vi "_PC_RTLoop_ReadLaserStatus.vi"(8 "error in (no error)":errorcluster, 9 "LaserStatus_string_reference in":refnum<vi>, 10 "Laser Status byte":refnum<vi>, 11 "stopRefnum":refnum<vi>) -> (0 "error out":errorcluster)   [LabVIEW 2018]
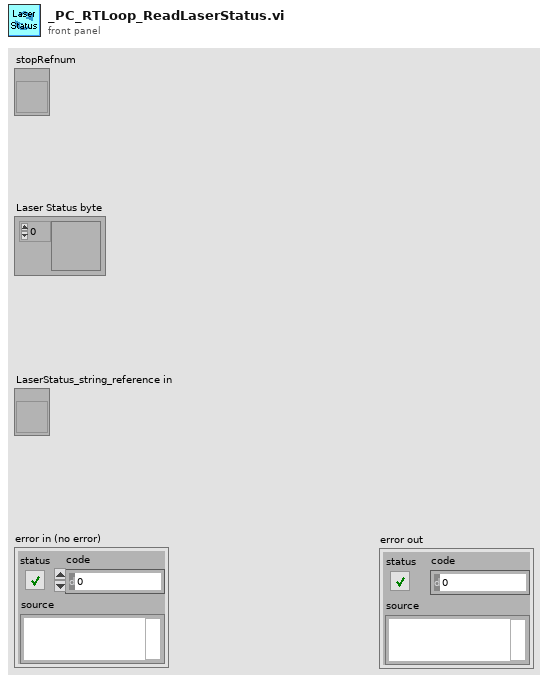
[diagram p1: front panel]
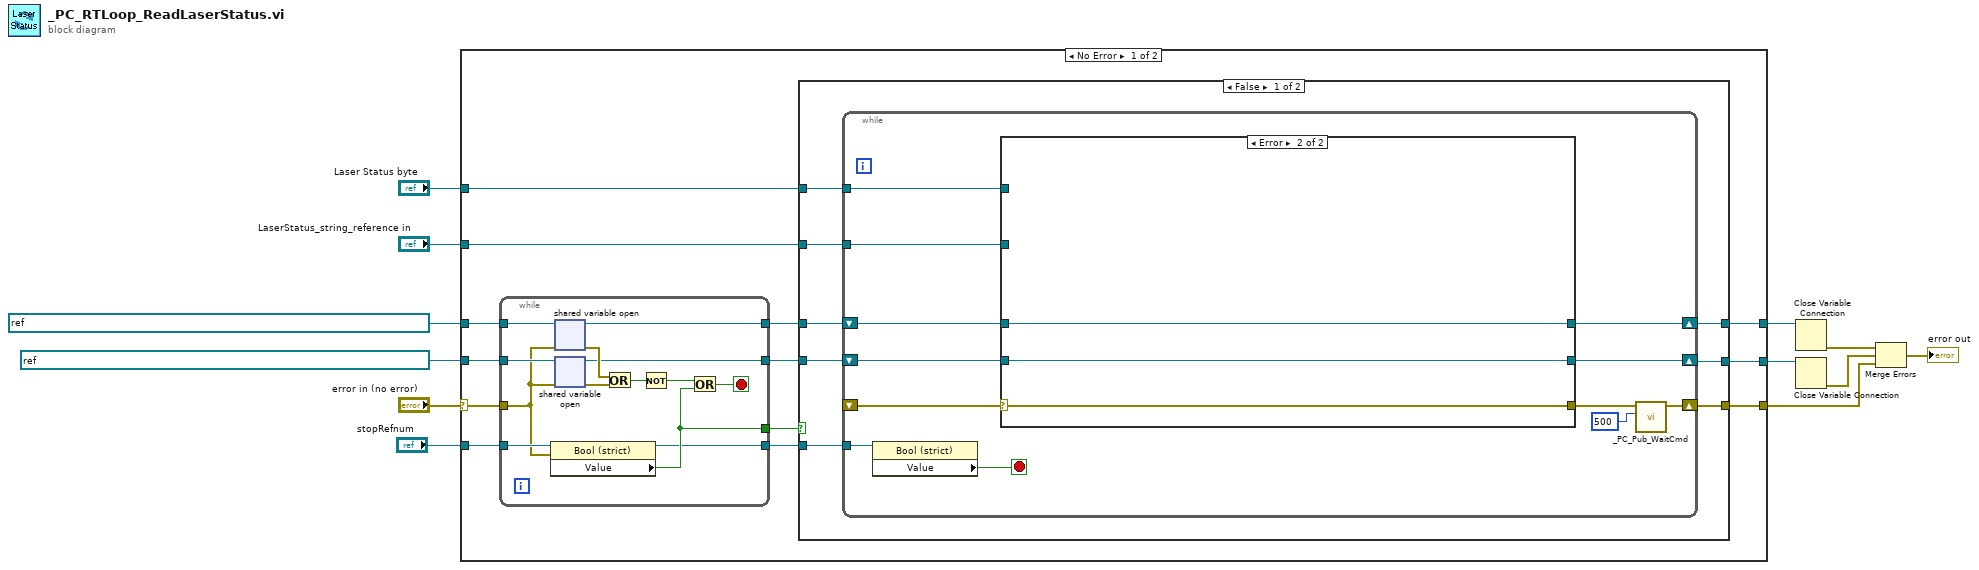
[diagram p0: block diagram]
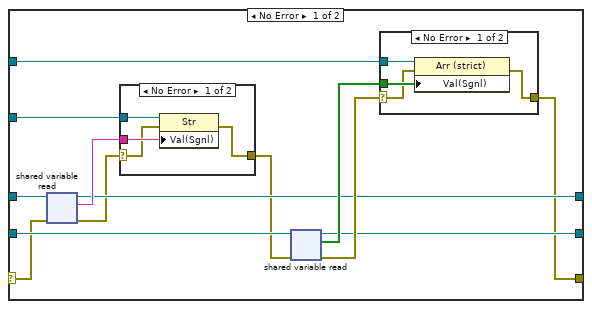
[diagram p2: hidden frame]
diagram:
  n1 = case shown="No Error" "error in (no error)" {
    selector: "error in (no error)" -> [w23 w87]
    tunnel: refnum<k21> "ni.var.psp://NI-sbRIO/_RT_CtrlLoop_Laser_Variables/LaserStatus_string" ("shared variable refnum in") -> [w25 w89]
    tunnel: refnum<k21> "ni.var.psp://NI-sbRIO/_RT_CtrlLoop_Laser_Variables/LaserStatusByte" ("shared variable refnum in") -> [w24 w88]
    tunnel: "LaserStatus_string_reference in" -> [w20 _]
    tunnel: "Laser Status byte" -> [w19 _]
    tunnel: [w18 w89] -> w7
    tunnel: [w17 w88] -> w6
    tunnel: "stopRefnum" -> [w16 _]
    tunnel: [w13 w87] -> w2
    frame No Error {
      n2 = while {
        tunnel: w25 -> [w86]
        tunnel: w24 -> [w85]
        tunnel: w23 -> [w74]
        tunnel: [w81] -> w21
        tunnel: [w80] -> w22
        tunnel: w16 -> [w77]
        tunnel: [w76] -> w14
        tunnel: [w75] -> w15
        stop <- w78 stop-if-true
        n3 = property class="Bool (strict)"(reference=w77, error in=w74) -> (reference out=w75:refnum<vi>, "Value"=w76:bool)  [unwired: 1 out]
        n4 = shared-variable-open(w86, w74) -> (w80:refnum<k21>, w84:errorcluster)
        n5 = shared-variable-open(w85, w74) -> (w81:refnum<k21>, w83:errorcluster)
        n6 = Or(x=w84, y=w83) -> (x .or. y?=w82:bool)
        n7 = Not(x=w82) -> (.not. x?=w79:bool)
        n8 = Or(x=w79, y=w76) -> (x .or. y?=w78:bool)
      }
      n9 = case shown="False" w14 {
        tunnel: w22 -> [w33 w73]
        tunnel: w21 -> [w32 w72]
        tunnel: w20 -> [w31 _]
        tunnel: w19 -> [w30 _]
        tunnel: [w29 w73] -> w18
        tunnel: [w28 w72] -> w17
        tunnel: w15 -> [w27 _]
        tunnel: [w26 _] -> w13
        frame False {
          n10 = while {
            tunnel: w31 -> [w43]
            tunnel: w30 -> [w42]
            tunnel: w27 -> [w35]
            shift-right: [w41] -> w29
            shift-left: w33 -> [w45]
            shift-right: [w40] -> w28
            shift-left: w32 -> [w44]
            shift-right: [w38] -> w26
            shift-left: _ -> [w36]
            stop <- w34 stop-if-true
            n11 = property class="Bool (strict)"(reference=w35) -> ("Value"=w34:bool)  [unwired: 1 in, 2 out]
            n12 = case shown="Error" w36 {
              selector: w36 -> [w46 w71]
              tunnel: w45 -> [w58 w69]
              tunnel: w44 -> [w57 w70]
              tunnel: w43 -> [w55 _]
              tunnel: w42 -> [w52 _]
              tunnel: [w51 w69] -> w41
              tunnel: [w50 w70] -> w40
              tunnel: [w47 w71] -> w39
              frame No Error {
                n13 = shared-variable-read(w58, w46) -> (w51:refnum<k21>, w49:errorcluster, w56:string)
                n14 = case shown="No Error" w49 {
                  selector: w49 -> [w65 w68]
                  tunnel: w55 -> [w67 _]
                  tunnel: w56 -> [w66 _]
                  tunnel: [w64 w68] -> w48
                  frame No Error {
                    n15 = property class="Str"(reference=w67, error in=w65, "Val(Sgnl)"=w66) -> (error out=w64:errorcluster)  [unwired: 1 out]
                  }
                  frame Error {
                  }
                }
                n16 = shared-variable-read(w57, w48) -> (w50:refnum<k21>, w53:errorcluster, w54:bool[])
                n17 = case shown="No Error" w53 {
                  selector: w53 -> [w60 w63]
                  tunnel: w52 -> [w62 _]
                  tunnel: w54 -> [w61 _]
                  tunnel: [w59 w63] -> w47
                  frame No Error {
                    n18 = property class="Arr (strict)"(reference=w62, error in=w60, "Val(Sgnl)"=w61) -> (error out=w59:errorcluster)  [unwired: 1 out]
                  }
                  frame Error {
                  }
                }
              }
              frame Error {
              }
            }
            n19 = call "_PC_Pub_WaitCmd.vi"("milliseconds to wait"=u32 500, "error in (no error)"=w39) -> ("error out"=w38:errorcluster)  [unwired: 9 in]
          }
        }
        frame True {
        }
      }
    }
    frame Error {
    }
  }
  n20 = Close Variable Connection(11:w7) -> (0:w5:errorcluster)  [unwired: 1 in]
  n21 = Close Variable Connection(11:w6) -> (0:w4:errorcluster)  [unwired: 1 in]
  n22 = Merge Errors(w5, w4, w2) -> (→"error out":errorcluster)
